vi "Set Port Status.vi"(8 "error in (no error)":errorcluster, 9 "Value":string, 10 "Port":dbl, 11 "Simulado in":refnum<class "Simulado.lvclass">) -> (0 "error out":errorcluster, 3 "Simulado out":refnum<class "Simulado.lvclass">)   [LabVIEW 2020, in "Simulado.lvclass"]
uses:
  Simulado.lvclass
  Simulado.lvclass/Simulado.ctl
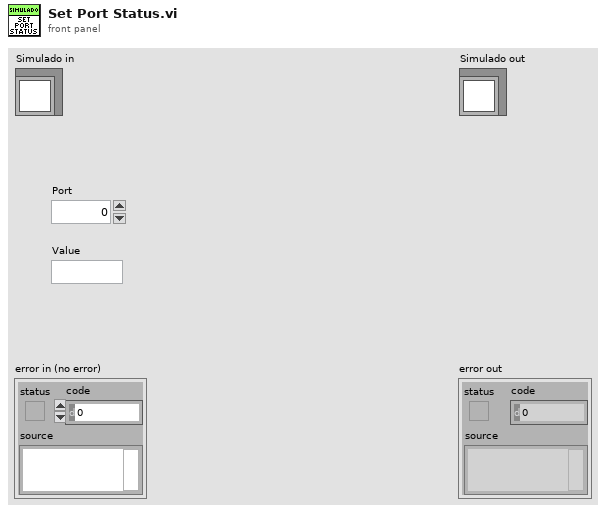
[diagram p1: front panel]
types:
  T1 = typedef "Serial device.lvclass/Brand combobox.ctl" = string
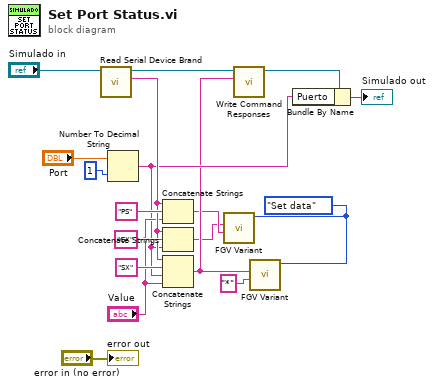
[diagram p0: block diagram]
diagram:
  w1 = enum16{"Reset data", "Set data", "Get data"}."Set data" ("Functions")
  n1 = call-dynamic "Read Serial Device Brand.vi"("Serial device in"="Simulado in") -> ("Serial Device Brand"=w12:T1, "Serial device out"=w11:refnum<class "Simulado.lvclass">)  [unwired: 8 in, 1 out]
  n2 = Number To Decimal String(number="Port", width (-)=i16 1) -> (decimal integer string=w6:string)
  n3 = Concatenate Strings(w12, "PS" ("string"), "Value") -> (w3:string)
  n4 = Concatenate Strings(w12, "GX" ("string"), w6) -> (w2:string)
  n5 = Concatenate Strings(w12, "SX" ("string"), w6, "Value") -> (w5:string)
  n6 = call "FGV Variant.vi"("Response to save"=w3, "Command"=w2, "Functions"=w1) -> ()  [unwired: 7 in, 2 out]
  n7 = call-dynamic "Write Command Responses.vi"("Command Responses"=w5, "Simulado in"=w11) -> ("Simulado out"=w10:refnum<class "Simulado.lvclass">)  [unwired: 8 in, 1 out]
  n8 = call "FGV Variant.vi"("Response to save"="*", "Command"=w5, "Functions"=w1) -> ()  [unwired: 7 in, 2 out]
  n9 = Bundle By Name(cluster=w10, "Puerto"=w6) -> (→"Simulado out":refnum<class "Simulado.lvclass">)
  "error out" <- "error in (no error)"
